vi "Command Interpreter.vi"(8 "error in (no error)":errorcluster) -> (0 "error out":errorcluster)   [LabVIEW 2016]
doc: "Provides command and control over the MyRIO via a command stream interface."
uses:
  RTLSDR Control/RTLSDR Global Variables.vi
  FPGA Control/FPGA Global Variables.vi
  <vilib>/Utility/error.llb/Error Cluster From Error Code.vi
  <vilib>/rvi/errors/niLvFpgaAdjustHostInterfaceError.vi
  <vilib>/rvi/interface/nirviReadWriteControl/nirviReadWriteControl.xnode
  <vilib>/rtlsdr/rtlsdr.lvlib
  NiFpgaLv.dll
  <vilib>/rvi/interface/Simulation/niFpgaSimulationCallBeginRW.vi
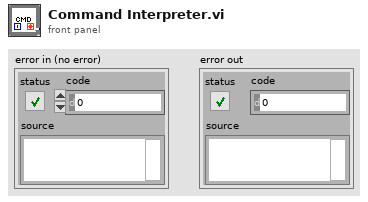
[diagram p1: front panel]
types:
  T1 = typedef "Command and Parameters.ctl" = cluster{"Command":T2, "Command Parameters":variant[]}
  T2 = typedef "Commands.ctl" = enum16{"Set Center Frequency", "Set AGC State", "Set Number Of Averages", "Set Tuner Gain Mode", "Set Frequency Correction", "Set Sample Rate", "Set Manual Gain Value"}
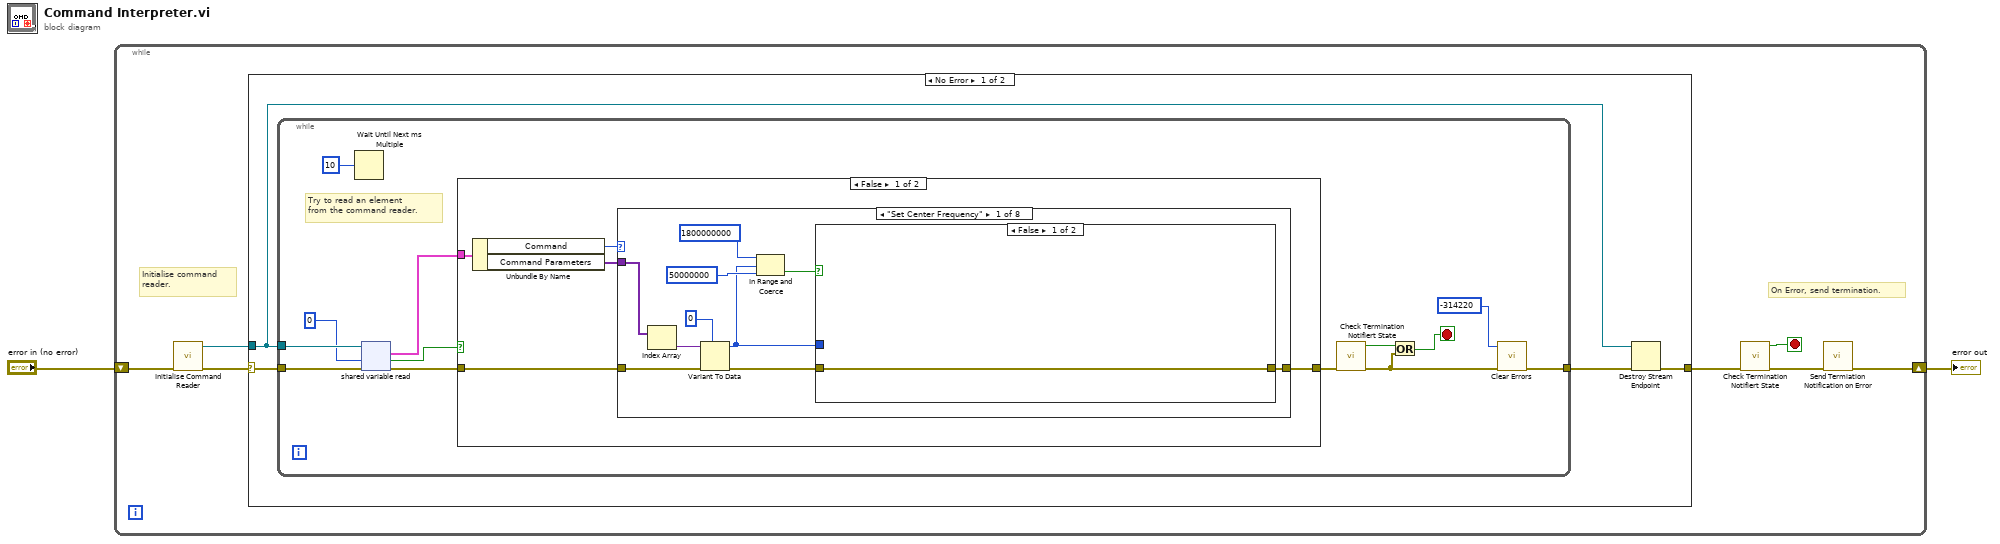
[diagram p0: block diagram]
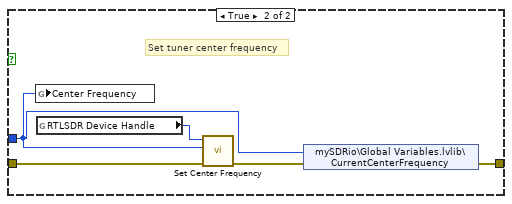
[diagram p2: hidden frame]
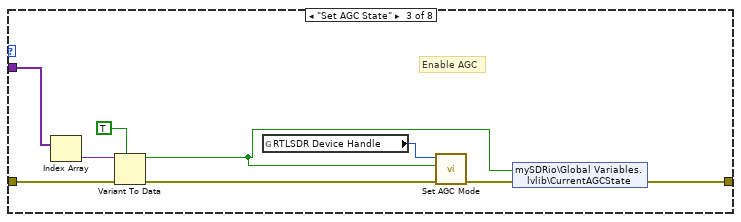
[diagram p4: hidden frame]
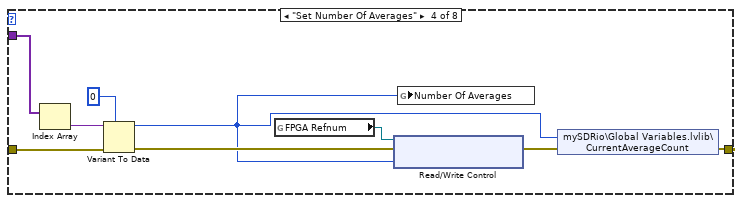
[diagram p5: hidden frame]
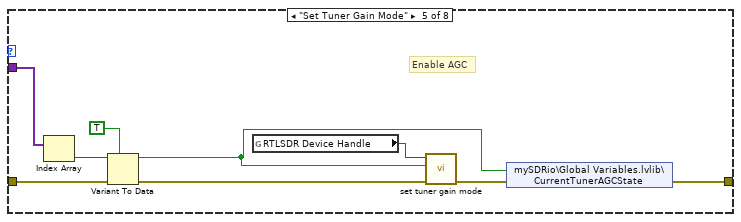
[diagram p6: hidden frame]
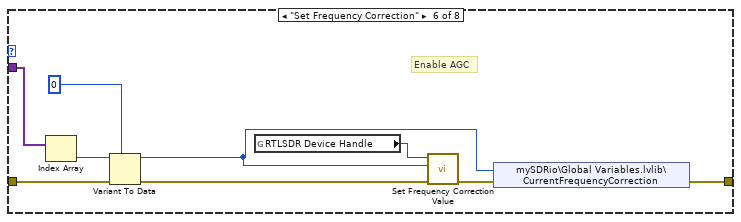
[diagram p7: hidden frame]
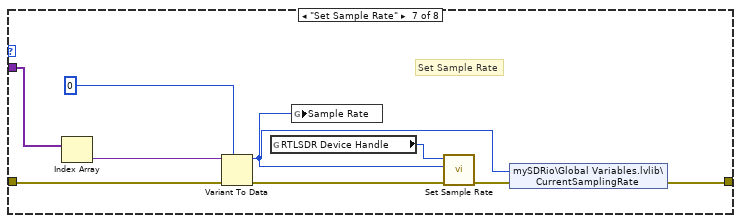
[diagram p8: hidden frame]
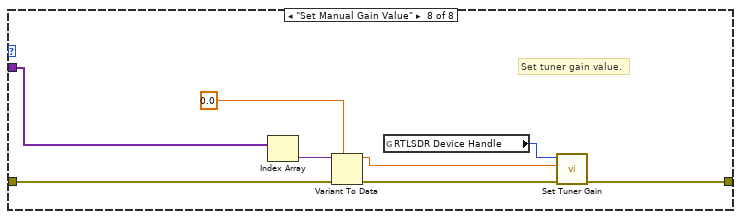
[diagram p9: hidden frame]
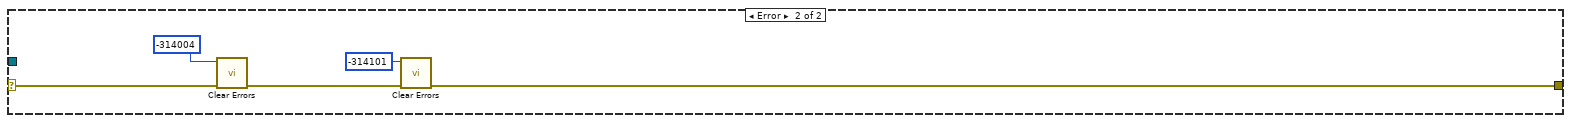
[diagram p11: hidden frame]
diagram:
  n1 = while {
    shift-right: [w7] -> w1
    shift-left: "error in (no error)" -> [w6]
    stop <- w8 stop-if-true
    # "Initialise command\nreader."
    # "On Error, send termination."
    n2 = call "Initialise Command Reader.vi"("error in (no error)"=w6) -> ("error out"=w5:errorcluster, "Refnum out"=w3:refnum<k21>)  [unwired: 9 in]
    n3 = case shown="No Error" w5 {
      selector: w5 -> [w13 w104]
      tunnel: [w11 w103] -> w4
      tunnel: w3 -> [w10 _]
      frame No Error {
        n4 = while {
          tunnel: [w25] -> w12
          tunnel: w13 -> [w21]
          tunnel: w10 -> [w20]
          stop <- w24 stop-if-true
          # "Try to read an element\nfrom the command reader."
          n5 = Wait Until Next ms Multiple(millisecond multiple=u32 10) -> ()  [unwired: 1 out]
          n6 = shared-variable-read(w20, w21, 0 ("timeout ms (-1)")) -> (w15:errorcluster, w18:bool, w17:T1)  [unwired: 1 out]
          n7 = case shown="False" w18 {
            tunnel: w17 -> [w31 _]
            tunnel: [w28 w102] -> w16
            tunnel: w15 -> [w29 w102]
            frame False {
              n8 = Unbundle By Name(w31) -> ("Command"=w30:T2, "Command Parameters"=w27:variant[])
              n9 = case shown="\"Set Center Frequency\"" w30 {
                tunnel: w29 -> [w38 w48 w55 w64 w71 w81 w88 w98]
                tunnel: [w36 w48 w50 w59 w68 w77 w86 w94] -> w28
                tunnel: w27 -> [w41 _ w53 w63 w70 w80 w87 w97]
                frame "Set Center Frequency" {
                  n10 = Index Array(array=w41) -> (element=w40:variant)  [unwired: 1 in]
                  n11 = Variant To Data(error in=w38, type=u32 0 ("Center Frequency"), Variant=w40) -> (data=w32:u32, error out=w37:errorcluster)
                  n12 = In Range and Coerce(upper limit=u32 1800000000, x=w32, lower limit=u32 50000000) -> (In Range?=w33:bool)  [unwired: 1 out]
                  n13 = case shown="False" w33 {
                    tunnel: w37 -> [w42 w46]
                    tunnel: [w42 w44] -> w36
                    tunnel: w32 -> [_ w43]
                    frame False {
                    }
                    frame True {
                      # "Set tuner center frequency"
                      n14 = global write "RTLSDR Global Variables.vi" "Center Frequency"(w43) -> ()
                      n15 = global read "RTLSDR Global Variables.vi" "RTLSDR Device Handle"() -> (w47:u64)
                      n16 = call "Set Center Frequency.vi"("error in (no error)"=w46, "Center Frequency"=w43, "DeviceRefnum"=w47) -> ("error out"=w45:errorcluster)  [unwired: 6 in, 2 out]
                      n17 = shared-variable "mySDRio\\Global Variables.lvlib\\CurrentCenterFrequency"(w43, error in=w45) -> (error out=w44:errorcluster)
                    }
                  }
                }
                frame Default {
                  # "Do nothing.  Default case."
                }
                frame "Set AGC State" {
                  # "Enable AGC"
                  n18 = Index Array(array=w53) -> (element=w57:variant)  [unwired: 1 in]
                  n19 = Variant To Data(error in=w55, type=TRUE, Variant=w57) -> (data=w49:bool, error out=w54:errorcluster)
                  n20 = global read "RTLSDR Global Variables.vi" "RTLSDR Device Handle"() -> (w52:u64)
                  n21 = call "Set AGC Mode.vi"("error in (no error)"=w54, "AGC Enable"=w49, "DeviceRefnum"=w52) -> ("error out"=w51:errorcluster)  [unwired: 6 in, 2 out]
                  n22 = shared-variable "mySDRio\\Global Variables.lvlib\\CurrentAGCState"(w49, error in=w51) -> (error out=w50:errorcluster)
                }
                frame "Set Number Of Averages" {
                  n23 = Index Array(array=w63) -> (element=w66:variant)  [unwired: 1 in]
                  n24 = Variant To Data(error in=w64, type=u32 0 ("Center Frequency"), Variant=w66) -> (data=w58:u32, error out=w62:errorcluster)
                  n25 = global read "FPGA Global Variables.vi" "FPGA Refnum"() -> (w61:refnum<k20>)
                  n26 = xnode "Read/Write Control"("FPGA VI Reference In"=w61, "error in"=w62, "Number Of Averages"=w58) -> ("error out"=w60:errorcluster)  [unwired: 1 out]
                  n27 = global write "FPGA Global Variables.vi" "Number Of Averages"(w58) -> ()
                  n28 = shared-variable "mySDRio\\Global Variables.lvlib\\CurrentAverageCount"(w58, error in=w60) -> (error out=w59:errorcluster)
                }
                frame "Set Tuner Gain Mode" {
                  # "Enable AGC"
                  n29 = Index Array(array=w70) -> (element=w75:variant)  [unwired: 1 in]
                  n30 = Variant To Data(error in=w71, type=TRUE, Variant=w75) -> (data=w67:bool, error out=w73:errorcluster)
                  n31 = global read "RTLSDR Global Variables.vi" "RTLSDR Device Handle"() -> (w72:u64)
                  n32 = call <vilib>:"set tuner gain mode.vi"("error in (no error)"=w73, "AutoGain"=w67, "DeviceRefnum"=w72) -> ("error out"=w69:errorcluster)  [unwired: 6 in, 2 out]
                  n33 = shared-variable "mySDRio\\Global Variables.lvlib\\CurrentTunerAGCState"(w67, error in=w69) -> (error out=w68:errorcluster)
                }
                frame "Set Frequency Correction" {
                  # "Enable AGC"
                  n34 = Index Array(array=w80) -> (element=w84:variant)  [unwired: 1 in]
                  n35 = Variant To Data(error in=w81, type=0, Variant=w84) -> (data=w76:i32, error out=w83:errorcluster)
                  n36 = global read "RTLSDR Global Variables.vi" "RTLSDR Device Handle"() -> (w82:u64)
                  n37 = call "Set Frequency Correction Value.vi"("error in (no error)"=w83, "Frequency Correction (ppm)"=w76, "DeviceRefnum"=w82) -> ("error out"=w78:errorcluster)  [unwired: 6 in, 2 out]
                  n38 = shared-variable "mySDRio\\Global Variables.lvlib\\CurrentFrequencyCorrection"(w76, error in=w78) -> (error out=w77:errorcluster)
                }
                frame "Set Sample Rate" {
                  # "Set Sample Rate"
                  n39 = Index Array(array=w87) -> (element=w93:variant)  [unwired: 1 in]
                  n40 = Variant To Data(error in=w88, type=u32 0, Variant=w93) -> (data=w85:u32, error out=w92:errorcluster)
                  n41 = global read "RTLSDR Global Variables.vi" "RTLSDR Device Handle"() -> (w91:u64)
                  n42 = global write "RTLSDR Global Variables.vi" "Sample Rate"(w85) -> ()
                  n43 = call "Set Sample Rate.vi"("error in (no error)"=w92, "Sample Rate"=w85, "DeviceRefnum"=w91) -> ("error out"=w89:errorcluster)  [unwired: 6 in, 2 out]
                  n44 = shared-variable "mySDRio\\Global Variables.lvlib\\CurrentSamplingRate"(w85, error in=w89) -> (error out=w86:errorcluster)
                }
                frame "Set Manual Gain Value" {
                  # "Set tuner gain value."
                  n45 = Index Array(array=w97) -> (element=w101:variant)  [unwired: 1 in]
                  n46 = Variant To Data(error in=w98, type=0.0, Variant=w101) -> (data=w95:dbl, error out=w100:errorcluster)
                  n47 = global read "RTLSDR Global Variables.vi" "RTLSDR Device Handle"() -> (w99:u64)
                  n48 = call "Set Tuner Gain.vi"("error in (no error)"=w100, "Gain (dB)"=w95, "DeviceRefnum"=w99) -> ("error out"=w94:errorcluster)  [unwired: 6 in, 2 out]
                }
              }
            }
            frame True {
            }
          }
          n49 = call "Check Termination Notifiert State.vi"("error in (no error)"=w16) -> ("error out"=w22:errorcluster, "Termination Notifier State"=w23:bool)  [unwired: 9 in]
          n50 = Or(x=w23, y=w22) -> (x .or. y?=w24:bool)
          n51 = call <vilib>:"Clear Errors.vi"("error in (no error)"=w22, "specific error code to clear (0: all)"=-314220) -> ("error out"=w25:errorcluster)  [unwired: 4 in, 1 out]
        }
        n52 = Destroy Stream Endpoint(8:w12, 11:w10) -> (0:w11:errorcluster)
      }
      frame Error {
        n53 = call <vilib>:"Clear Errors.vi"("error in (no error)"=w104, "specific error code to clear (0: all)"=-314004 ("y")) -> ("error out"=w106:errorcluster)  [unwired: 4 in, 1 out]
        n54 = call <vilib>:"Clear Errors.vi"("error in (no error)"=w106, "specific error code to clear (0: all)"=-314101) -> ("error out"=w103:errorcluster)  [unwired: 4 in, 1 out]
      }
    }
    n55 = call "Check Termination Notifiert State.vi"("error in (no error)"=w4) -> ("error out"=w9:errorcluster, "Termination Notifier State"=w8:bool)  [unwired: 9 in]
    n56 = call "Send Termiation Notification on Error.vi"("error in (no error)"=w9) -> ("error out"=w7:errorcluster)  [unwired: 10 in]
  }
  "error out" <- w1
